vi "Convert 2D to 1D Boolean.vi"(11 "2D Array":bool[][](array[boolean])) -> (1 "size(s)":i32[](array[numeric]), 3 "1D Array":bool[](array[boolean]))   [LabVIEW 2014]
doc: "<B>Copyright</B>: (c) MHWirth 2015. All rights reserved.\n\nThis subVI reshapes the input 2D array to 1D array."
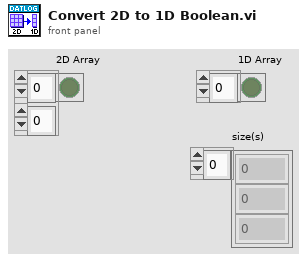
[diagram p1: front panel]
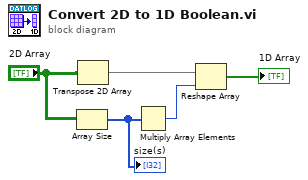
[diagram p0: block diagram]
diagram:
  n1 = Array Size(array="2D Array") -> (size(s)=w5:i32[])
  "size(s)" <- w5
  n2 = Transpose 2D Array(2D array="2D Array") -> (transposed array=w3:bool[][])
  n3 = Multiply Array Elements(1:w5) -> (0:w2:i32)
  n4 = Reshape Array(w3, w2) -> (→"1D Array":bool[])
